vi "Get File Name or Folder Name (wo .ext).vi"(8 "error in (no error)":errorcluster, 11 "input path":path) -> (0 "error out":errorcluster, 2 "filename without extension":string, 3 "dup path":path)   [LabVIEW 2021, in "Files.lvlib"]
uses:
  Files.lvlib
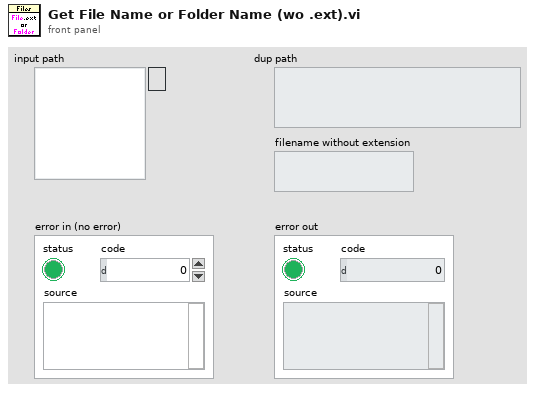
[diagram p1: front panel]
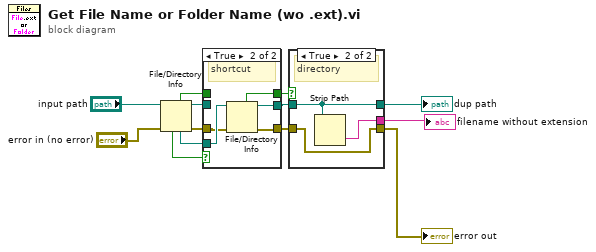
[diagram p0: block diagram]
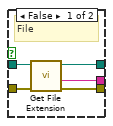
[diagram p2: hidden frame]
diagram:
  n1 = File/Directory Info(path="input path", error in="error in (no error)") -> (path out=w5:path, directory=w6:bool, error out=w4:errorcluster, resolved path=w7:path, shortcut=w8:bool)  [unwired: 2 out]
  n2 = case shown="True" w8 {
    tunnel: w7 -> [_ w21]
    tunnel: [w15 w20] -> w1
    tunnel: [w16 w19] -> w2
    tunnel: w6 -> [w16 _]
    tunnel: w5 -> [w15 _]
    tunnel: w4 -> [w14 w17]
    tunnel: [w14 w18] -> w3
    frame False {
    }
    frame True {
      # "shortcut"
      n3 = File/Directory Info(path=w21, error in=w17) -> (path out=w20:path, directory=w19:bool, error out=w18:errorcluster)  [unwired: 4 out]
    }
  }
  n4 = case shown="True" w2 {
    tunnel: [w26 w27] -> w13
    tunnel: [w25 w28] -> w12
    tunnel: [w24 w29] -> w11
    tunnel: w3 -> [w23 w27]
    tunnel: w1 -> [w22 w29]
    frame False {
      # "File"
      n5 = call <vilib>:"Get File Extension.vi"("error in (no error)"=w23, "file"=w22) -> ("error out"=w26:errorcluster, "filename without extension"=w25:string, "dup file"=w24:path)  [unwired: 5 in, 2 out]
    }
    frame True {
      # "directory"
      n6 = Strip Path(path=w29) -> (name=w28:string)  [unwired: 1 out]
    }
  }
  "error out" <- w13
  "filename without extension" <- w12
  "dup path" <- w11
